vi "Read Wavelength Test.vi"(3 "Error In (no error)":errorcluster, 5 "Resource Name":refnum<visa-resource-name>="ASRL1::INSTR") -> (0 "Error Out":errorcluster, 1 "Wavelength":dbl format="%.3f", 2 "Resource Name 2":refnum<visa-resource-name>="ASRL1::INSTR")   [LabVIEW 2017]
panel:
  out "Numeric":i32
  in  "Bytes to Read":u32=54
  out "Read Whole String":string
  in  "CW":string="CW"
  # "nm"
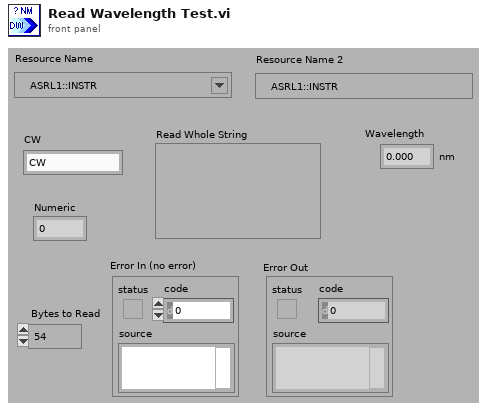
[diagram p1: front panel]
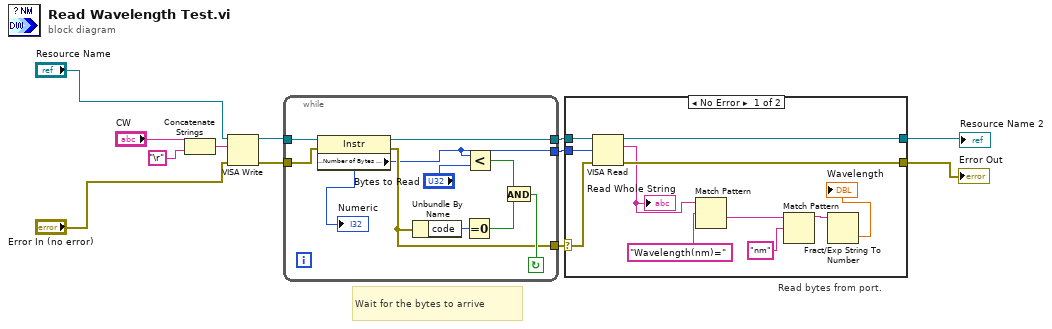
[diagram p0: block diagram]
diagram:
  # "Wait for the bytes to arrive"
  n1 = Concatenate Strings("CW", "\r") -> (w12:string)
  n2 = VISA Write(VISA resource name="Resource Name", write buffer=w12, error in (no error)="Error In (no error)") -> (VISA resource name out=w2:refnum<visa-resource-name>, error out=w1:errorcluster)  [unwired: 1 out]
  n3 = while {
    tunnel: [w15] -> w7
    tunnel: [w13] -> w8
    tunnel: w2 -> [w21]
    tunnel: w1 -> [w16]
    tunnel: [w22] -> w9
    stop <- w18 continue-if-true
    n4 = property class="Instr"(reference=w21, error in=w16) -> (reference out=w22:refnum<visa-resource-name>, error out=w15:errorcluster, "Serial Settings:Number of Bytes at Serial Port"=w13:u32)
    "Numeric" <- w13
    n5 = Unbundle By Name(w15) -> ("code"=w17:i32)
    n6 = Equal To 0?(x=w17) -> (x = 0?=w19:bool)
    n7 = Less?(x=w13, y="Bytes to Read") -> (x < y?=w20:bool)
    n8 = And(x=w20, y=w19) -> (x .and. y?=w18:bool)
  }
  n9 = case "Read bytes from port." shown="No Error" w7 {
    selector: w7 -> [w30 w34]
    tunnel: [w33 w34] -> w5
    tunnel: w9 -> [w32 w35]
    tunnel: w8 -> [w31 _]
    tunnel: [w29 w35] -> w6
    frame No Error {
      n10 = VISA Read(VISA resource name=w32, byte count=w31, error in (no error)=w30) -> (VISA resource name out=w29:refnum<visa-resource-name>, read buffer=w26:string, error out=w33:errorcluster)  [unwired: 1 out]
      "Read Whole String" <- w26
      n11 = Match Pattern(string=w26, regular expression="Wavelength(nm)=") -> (after substring=w27:string)  [unwired: 1 in, 3 out]
      n12 = Match Pattern(string=w27, regular expression="nm") -> (before substring=w24:string)  [unwired: 1 in, 3 out]
      n13 = Fract/Exp String To Number(string=w24) -> (number=→"Wavelength":dbl)  [unwired: 3 in, 1 out]
    }
    frame Error {
      # "Error occurred \nreading Bytes at \nSerial Port"
    }
  }
  "Error Out" <- w5
  "Resource Name 2" <- w6
